vi "Main..LabSSH.vi"() -> ()   [LabVIEW 2016, in "labssh_thijs.lvlib" / "LabSSH.lvlib"]
uses:
  LabSSH.lvlib
  State..enum.ctl
  LabSSH/LabSSH/LabSSH/bin/Debug/State Date..cluster.ctl
  C:/Users/thosman/Documents/Development/Labview/ssh in labview/LabSSH/LabSSH/LabSSH/bin/Debug/LabSSH.dll
  LabSSH/LabSSH/LabSSH/bin/Debug/LabSSH.dll
  <vilib>/Utility/cursorutil.llb/Set Cursor (Icon Pict).vi
  C:/Users/thosman/Documents/Development/Labview/ssh in labview/LabSSH/LabSSH/References/Renci.SshNet.dll
  LabSSH/LabSSH/References/Renci.SshNet.dll
panel:
  out "error in (no error)":errorcluster
  in  "Password":string="raspberry"
  in  "User Name":string="pi"
  in  "Host Address":string="192.168.0.106"
  out "Output":string
  in  "Input":string
  in  "Execute":bool
  in  "Disconnect":bool
  in  "Connect":bool
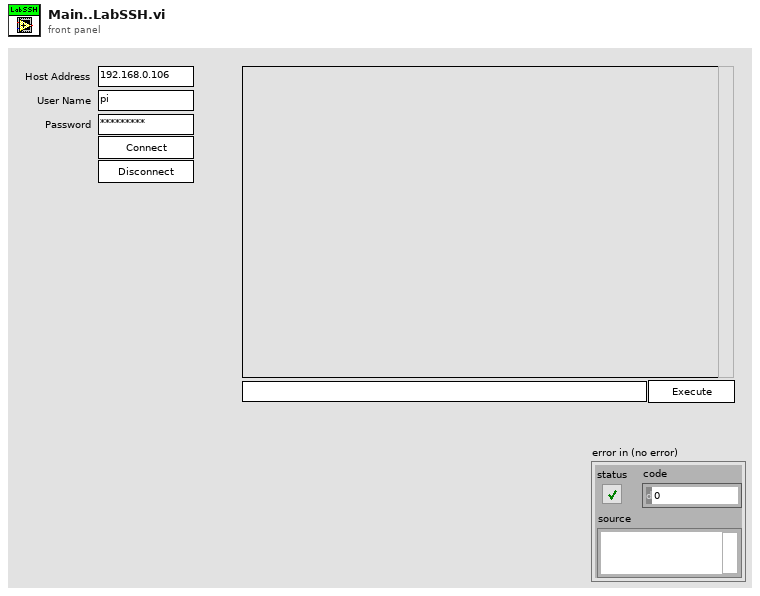
[diagram p1: front panel]
types:
  T1 = typedef "labssh_thijs.lvlib/LabSSH.lvlib/State Date..cluster.ctl" = cluster{"Object reference":refnum<k24>, "sshClient":refnum<k24>, "stream":refnum<k24>, "writer":refnum<k24>, "reader":refnum<k24>, "Output ref":refnum<vi>, "Timout (s)":i32}
  T2 = typedef "labssh_thijs.lvlib/LabSSH.lvlib/State..enum.ctl" = enum16{"", "Initialise", "Connect", "Execute Command", "Read Stream", "Disconnect", "Exit"}
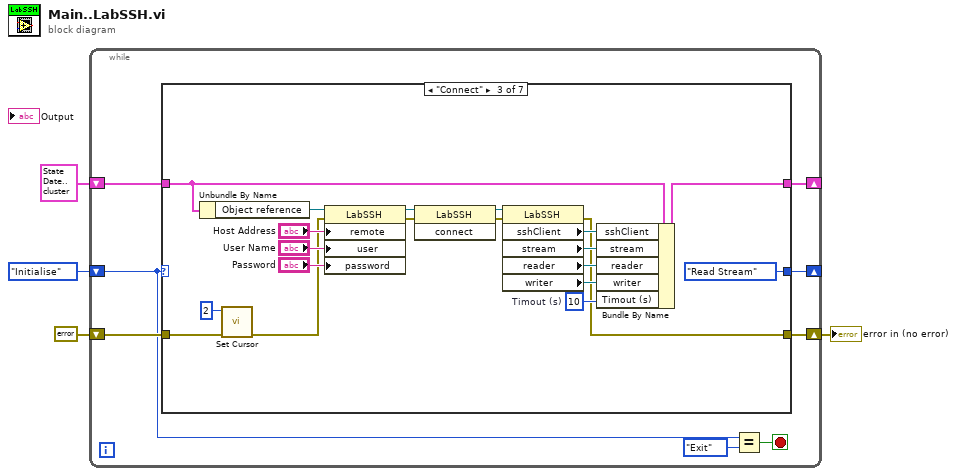
[diagram p0: block diagram]
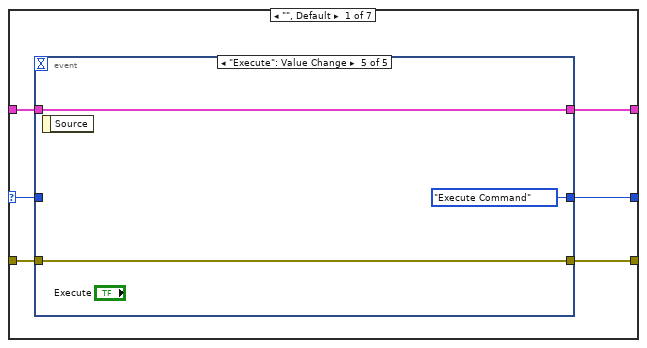
[diagram p2: hidden frame]
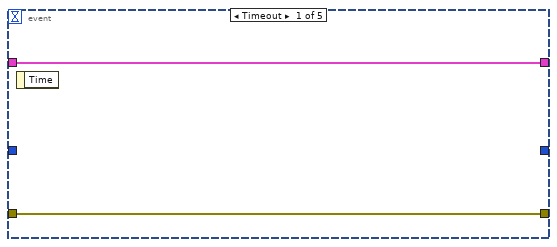
[diagram p3: hidden frame]
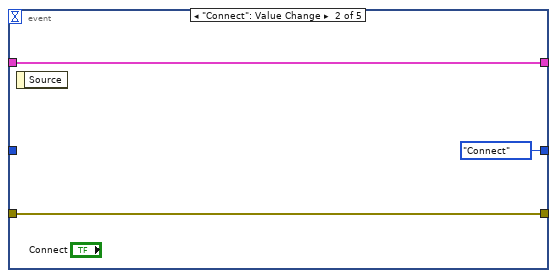
[diagram p4: hidden frame]
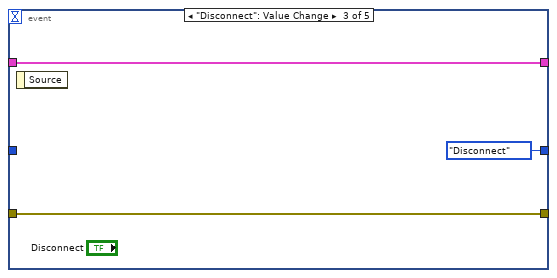
[diagram p5: hidden frame]
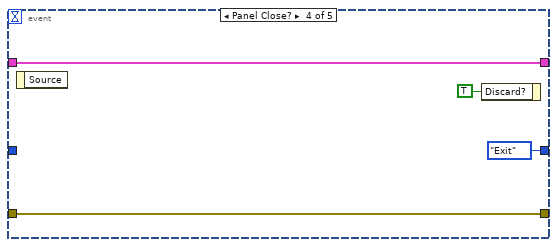
[diagram p6: hidden frame]
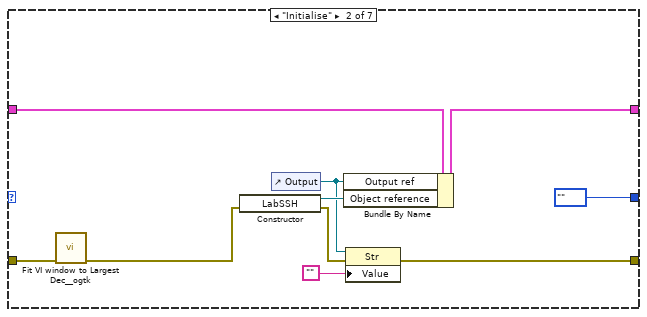
[diagram p7: hidden frame]
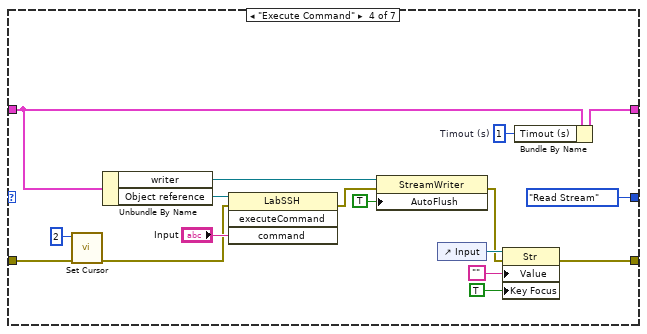
[diagram p8: hidden frame]
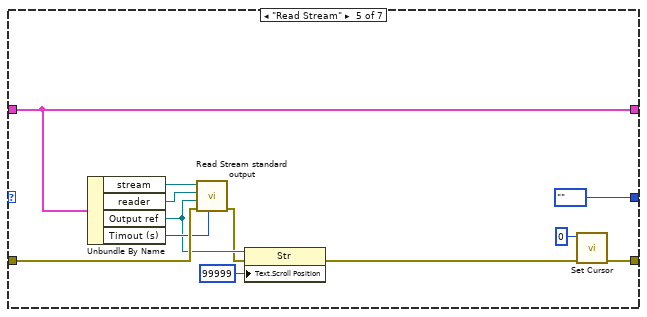
[diagram p9: hidden frame]
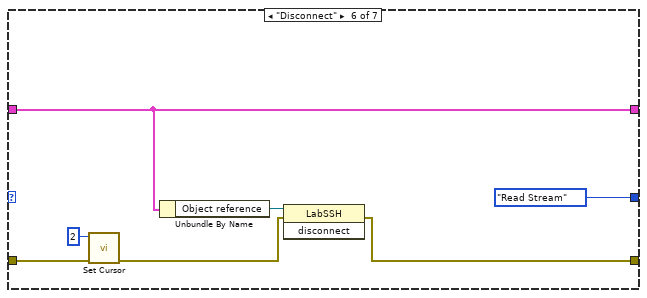
[diagram p10: hidden frame]
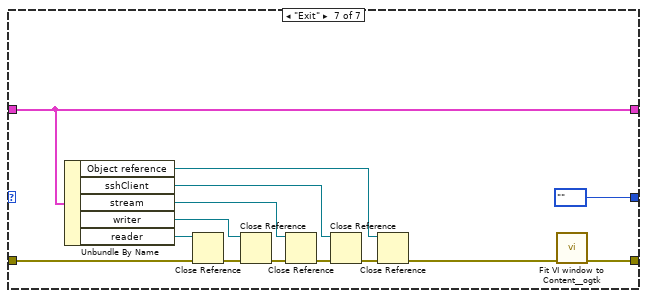
[diagram p11: hidden frame]
diagram:
  n1 = while {
    shift-right: [w12] -> _
    shift-left: State..enum."Initialise" -> [w7]
    shift-right: [w10] -> _
    shift-left: T1 {"Object reference"=refnum, "sshClient"=refnum, "stream"=refnum, "writer"=refnum, "reader"=refnum, "Output ref"=refnum, "Timout (s)"=0} -> [w11]
    shift-right: [w8] -> w2
    shift-left: errorcluster {"status"=FALSE, "code"=0, "source"=""} ("error in (no error)") -> [w9]
    stop <- w5 stop-if-true
    n2 = case shown="\"Connect\"" w7 {
      selector: w7 -> [w18 _ _ _ _ _ _]
      tunnel: [w17 State..enum."" State..enum."Read Stream" State..enum."Read Stream" State..enum."" State..enum."Read Stream" State..enum.""] -> w12
      tunnel: w11 -> [w16 w43 w63 w79 w91 w98 w111]
      tunnel: [w15 w42 w59 w73 w91 w98 w111] -> w10
      tunnel: w9 -> [w13 w38 w47 w65 w88 w94 w113]
      tunnel: [w14 w36 w44 w69 w83 w96 w100] -> w8
      frame "", Default {
        n3 = event shown="[4] \"Execute\": Value Change" {
          selector: _ -> [_ _ _ _ _]
          dyn-events: _ -> [_ _ _ _ _]
          timeout: _ -> [_ _ _ _ _]
          tunnel: w18 -> [_ _ _ _ _]
          tunnel: [_ State..enum."Connect" State..enum."Disconnect" State..enum."Exit" State..enum."Execute Command"] -> w17
          tunnel: [w20 w21 w26 w30 w33] -> w15
          tunnel: w16 -> [w20 w21 w26 w30 w33]
          tunnel: [w19 w23 w25 w29 w32] -> w14
          tunnel: w13 -> [w19 w23 w25 w29 w32]
          event Timeout {
            n4 = event-data() -> ()  [unwired: 1 in, 1 out]
          }
          event "Connect": Value Change {
            n5 = event-data() -> ()  [unwired: 1 in, 1 out]
          }
          event "Disconnect": Value Change {
            n6 = event-data() -> ()  [unwired: 1 in, 1 out]
          }
          event Panel Close? {
            n7 = event-data() -> ()  [unwired: 1 in, 1 out]
            n8 = event-data("Discard?"=TRUE) -> ()  [unwired: 1 in, 1 out]
          }
          event "Execute": Value Change {
            n9 = event-data() -> ()  [unwired: 1 in, 1 out]
          }
        }
      }
      frame "Initialise" {
        n10 = call <userlib>:"Fit VI window to Largest Dec__ogtk.vi"("error in (no error)"=w38) -> ("error out"=w37:errorcluster)  [unwired: 5 in, 1 out]
        n11 = constructor class="LabSSH"(error in=w37) -> (reference out=w41:refnum<k24>, error out=w40:errorcluster)  [unwired: 2 in, 1 out]
        n12 = control-ref of="Output"() -> (w35:refnum<vi>)
        n13 = Bundle By Name(cluster=w43, "Output ref"=w35, "Object reference"=w41) -> (w42:T1)
        n14 = property class="Str"(reference=w35, error in=w40, "Value"="") -> (error out=w36:errorcluster)  [unwired: 1 out]
      }
      frame "Connect" {
        w48 = 10  # Timout (s)
        n15 = Unbundle By Name(w63) -> ("Object reference"=w62:refnum<k24>)
        n16 = call-poly <vilib>:"Set Cursor.vi"("error in (no error)"=w47, "icon"=u16 2) -> ("error out"=w46:errorcluster)  [unwired: 8 in, 1 out]
        n17 = property class="LabSSH"(reference=w62, error in=w46, "remote"="Host Address", "user"="User Name", "password"="Password") -> (reference out=w53:refnum<k24>, error out=w52:errorcluster)
        n18 = invoke class="LabSSH" method="connect"(reference=w53, error in=w52) -> (reference out=w61:refnum<k24>, error out=w60:errorcluster)  [unwired: 1 in, 1 out]
        n19 = property class="LabSSH"(reference=w61, error in=w60) -> (error out=w44:errorcluster, "sshClient"=w58:refnum<k24>, "stream"=w57:refnum<k24>, "reader"=w56:refnum<k24>, "writer"=w55:refnum<k24>)  [unwired: 1 out]
        n20 = Bundle By Name(cluster=w63, "sshClient"=w58, "stream"=w57, "reader"=w56, "writer"=w55, "Timout (s)"=w48) -> (w59:T1)
      }
      frame "Execute Command" {
        w72 = 1  # Timout (s)
        n21 = call-poly <vilib>:"Set Cursor.vi"("error in (no error)"=w65, "icon"=u16 2) -> ("error out"=w64:errorcluster)  [unwired: 8 in, 1 out]
        n22 = Unbundle By Name(w79) -> ("writer"=w76:refnum<k24>, "Object reference"=w78:refnum<k24>)
        n23 = invoke class="LabSSH" method="executeCommand"(reference=w78, error in=w64, "command"="Input") -> (error out=w74:errorcluster)  [unwired: 1 in, 3 out]
        n24 = property class="StreamWriter"(reference=w76, error in=w74, "AutoFlush"=TRUE) -> (error out=w70:errorcluster)  [unwired: 1 out]
        n25 = control-ref of="Input"() -> (w71:refnum<vi>)
        n26 = property class="Str"(reference=w71, error in=w70, "Value"="", "Key Focus"=TRUE) -> (error out=w69:errorcluster)  [unwired: 1 out]
        n27 = Bundle By Name(cluster=w79, "Timout (s)"=w72) -> (w73:T1)
      }
      frame "Read Stream" {
        n28 = Unbundle By Name(w91) -> ("stream"=w90:refnum<k24>, "reader"=w89:refnum<k24>, "Output ref"=w86:refnum<vi>, "Timout (s)"=w87:i32)
        n29 = call "Read Stream standard output.vi"("Timout (s)"=w87, "error in (no error)"=w88, "Output ref"=w86, "reader"=w89, "stream"=w90) -> ("error out"=w82:errorcluster)  [unwired: 6 in]
        n30 = property class="Str"(reference=w86, error in=w82, "Text.Scroll Position"=u32 99999) -> (error out=w81:errorcluster)  [unwired: 1 out]
        n31 = call-poly <vilib>:"Set Cursor.vi"("error in (no error)"=w81, "icon"=u16 0) -> ("error out"=w83:errorcluster)  [unwired: 8 in, 1 out]
      }
      frame "Disconnect" {
        n32 = call-poly <vilib>:"Set Cursor.vi"("error in (no error)"=w94, "icon"=u16 2) -> ("error out"=w93:errorcluster)  [unwired: 8 in, 1 out]
        n33 = Unbundle By Name(w98) -> ("Object reference"=w97:refnum<k24>)
        n34 = invoke class="LabSSH" method="disconnect"(reference=w97, error in=w93) -> (error out=w96:errorcluster)  [unwired: 1 in, 2 out]
      }
      frame "Exit" {
        n35 = Unbundle By Name(w111) -> ("Object reference"=w102:refnum<k24>, "sshClient"=w103:refnum<k24>, "stream"=w104:refnum<k24>, "writer"=w105:refnum<k24>, "reader"=w106:refnum<k24>)
        n36 = Close Reference(reference=w106, error in (no error)=w113) -> (error out=w107:errorcluster)
        n37 = Close Reference(reference=w105, error in (no error)=w107) -> (error out=w110:errorcluster)
        n38 = Close Reference(reference=w104, error in (no error)=w110) -> (error out=w108:errorcluster)
        n39 = Close Reference(reference=w103, error in (no error)=w108) -> (error out=w109:errorcluster)
        n40 = Close Reference(reference=w102, error in (no error)=w109) -> (error out=w101:errorcluster)
        n41 = call <userlib>:"Fit VI window to Content__ogtk.vi"("error in (no error)"=w101) -> ("error out"=w100:errorcluster)  [unwired: 5 in, 1 out]
      }
    }
    n42 = Equal?(x=w7, y=State..enum."Exit") -> (x = y?=w5:bool)
  }
  "error in (no error)" <- w2
